vi "EXA shm get Event Heartbeat In LV.vi"(8 "error in (no error)":errorcluster, 11 "logevent_HeartbeatIn_Ctl":T1) -> (0 "error out":errorcluster, 2 "function return":i32, 3 "logevent_HeartbeatIn_Ctl out":T1)   [LabVIEW 2016, in "SALLV_EXA.lvlib"]
doc: "int EXA_shm_getEvent_HeartbeatInLV(EXA_logevent_HeartbeatInLV *logevent_HeartbeatIn_Ctl );"
uses:
  SALLV_EXA.lvlib
  SALLV_EXA.so
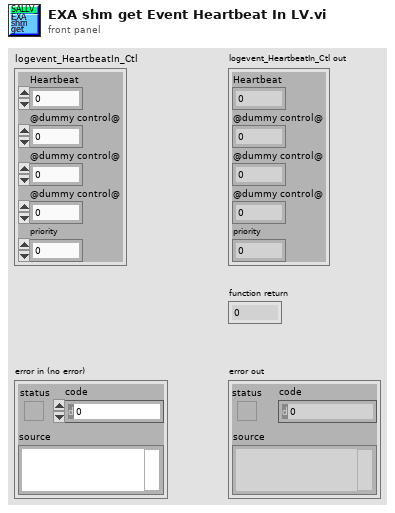
[diagram p1: front panel]
types:
  T1 = cluster{"Heartbeat":u8, "@dummy control@":i8, "@dummy control@":i8, "@dummy control@":i8, "priority":i32}
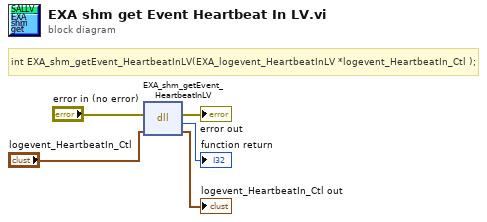
[diagram p0: block diagram]
diagram:
  # "int EXA_shm_getEvent_HeartbeatInLV(EXA_logevent_HeartbeatInLV *logevent_HeartbeatIn_Ctl );"
  n1 = dll-call lib="home/plotz/SALLV_EXA/SALLV_EXA.*" fn="EXA_shm_getEvent_HeartbeatInLV"(error in="error in (no error)", "logevent_HeartbeatIn_Ctl"="logevent_HeartbeatIn_Ctl") -> (error out=→"error out":errorcluster, →"function return":i32, "logevent_HeartbeatIn_Ctl"=→"logevent_HeartbeatIn_Ctl out":T1)  [unwired: 2 in, 1 out]
